vi "IPI_CCD_Write_Result.vi"(9 "Origin":cluster{"X":i32, "Y":i32}, 10 "Result":string, 11 "Image in":T1(plugin-control)) -> (3 "Image Out":T1(plugin-control))   [LabVIEW 2015]
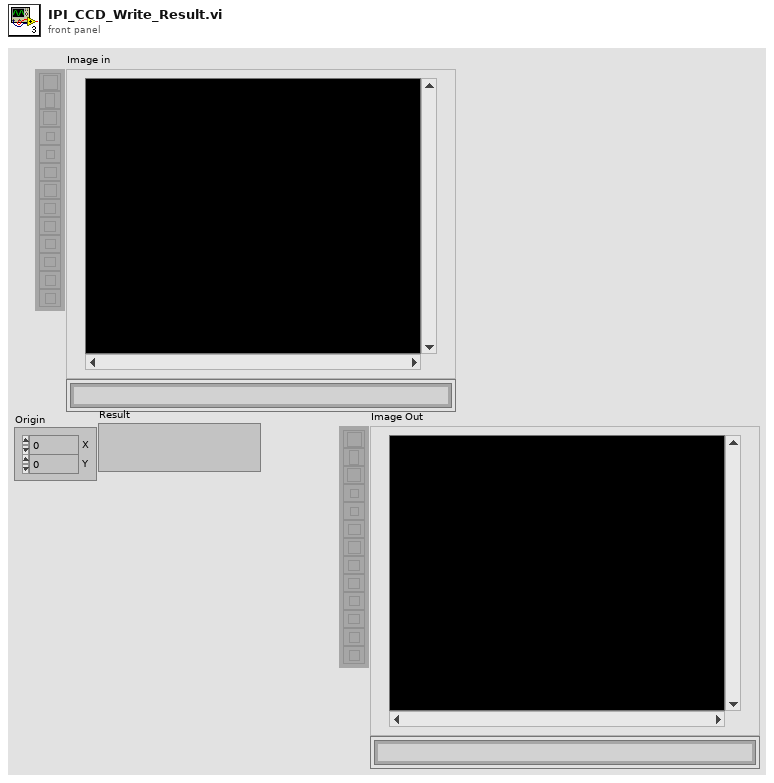
[diagram p1: front panel]
types:
  T1 = typedef "IMAQ Image.ctl" = refnum<image>
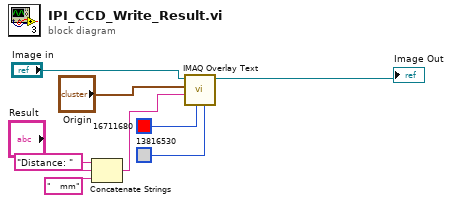
[diagram p0: block diagram]
diagram:
  n1 = Concatenate Strings("Distance: " ("字符串"), "Result", "   mm" ("字符串")) -> (w1:string)
  n2 = call "IMAQ Overlay Text"("BG Color (Transparent)"=u32 13816530, "Text Color (black)"=u32 16711680, "String"=w1, "Origin"="Origin", "Image"="Image in") -> ("Image Out"=→"Image Out":T1)  [unwired: 5 in, 1 out]
